vi "Set SshHostKeyPolicy.vi"(8 "error in (no error)":errorcluster, 10 "SshHostKeyPolicy":T1=1 items=["Check", "GiveUpSecurityAndAcceptAny", "AcceptNew"], 11 "SessionOptions-SCP in":refnum<class "SessionOptions-SCP.lvclass">) -> (0 "error out":errorcluster, 3 "SessionOptions-SCP out":refnum<class "SessionOptions-SCP.lvclass">)   [LabVIEW 2015, in "SessionOptions-SCP.lvclass"]
uses:
  SessionOptions-SCP.lvclass
  SSHHostKeyPolicy.ctl
  Protocols--Ring.ctl
  SessionOptions-SCP.lvclass/SessionOptions-SCP.ctl
  SessionOptions.lvclass
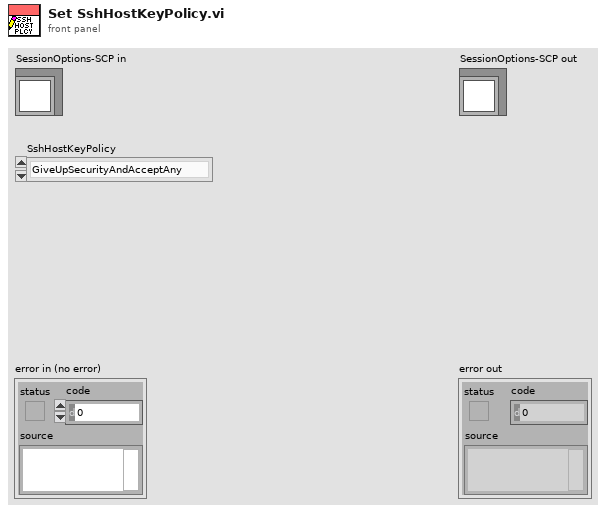
[diagram p1: front panel]
types:
  T1 = typedef "SessionOptions-SCP.lvclass/SSHHostKeyPolicy.ctl" = i32
  T2 = typedef "SessionOptions.lvclass/Protocols--Ring.ctl" = i32
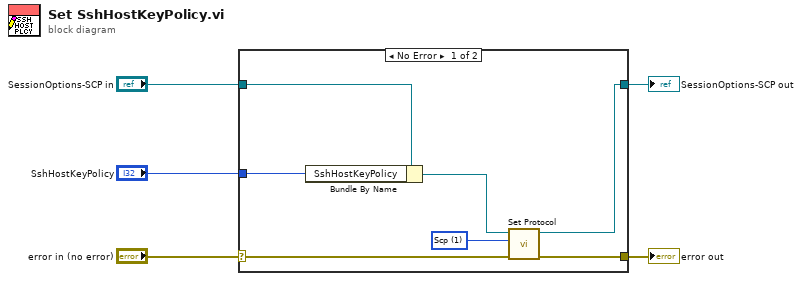
[diagram p0: block diagram]
diagram:
  n1 = case shown="No Error" "error in (no error)" {
    selector: "error in (no error)" -> [w8 w13]
    tunnel: [w7 w13] -> w4
    tunnel: [w9 w14] -> w2
    tunnel: "SessionOptions-SCP in" -> [w12 w14]
    tunnel: "SshHostKeyPolicy" -> [w11 _]
    frame No Error {
      w6 = T2 1 items=["Sftp", "Scp", "Ftp", "Webdav", "S3"] ("Protocol")
      n2 = Bundle By Name(cluster=w12, "SshHostKeyPolicy"=w11) -> (w10:refnum<class "SessionOptions-SCP.lvclass">)
      n3 = call "Set Protocol.vi"("error in (no error)"=w8, "Protocol"=w6, "SessionOptions in"=w10) -> ("error out"=w7:errorcluster, "SessionOptions out"=w9:refnum<class "SessionOptions-SCP.lvclass">)  [unwired: 7 in]
    }
    frame Error {
    }
  }
  "error out" <- w4
  "SessionOptions-SCP out" <- w2
